vi "Add Port RTM.vi"(8 "error in":errorcluster, 11 "Node Ptr":T1 format="%.0x") -> (0 "error out":errorcluster)   [LabVIEW 2020, in "Ballard ARINC 429 System Explorer.lvlib" / "Implementation.lvlib"]
doc: "This VI runs when the Add Port run-time menu is chosen. It allows the user to create a port with an associated database."
uses:
  Implementation.lvlib
  <vilib>/NI VeriStand/Custom Device Tools/Custom Device Utility Library/Custom Device Utility Library.lvlib
  <vilib>/NI VeriStand/Custom Device API/Custom Device Item Ref.ctl
  <vilib>/NI VeriStand/Custom Device API/Custom Device API.lvlib
  Scripting/Ballard ARINC 429 Scripting.lvlib
  Scripting/Constants.vi
panel:
  in  "Baud Rate":u32
  in  "Database":string(combo)
  in  "Port Name":string
  in  "Help":bool
  in  "Cancel":bool
  in  "OK":bool
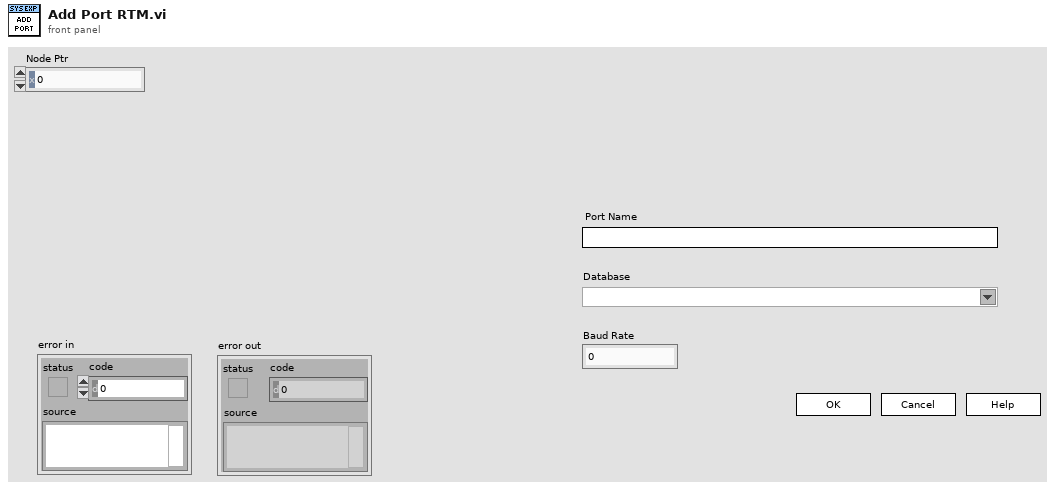
[diagram p1: front panel]
types:
  T1 = typedef "Custom Device API.lvlib/Custom Device Item Ref.ctl" = u64
  T2 = cluster{"Baud Rate":u32, "Port Name":string, "Database Name":string, "Database Path":path, "Databases ref":T1, "Node Ptr":T1}
  T3 = typedef "Ballard ARINC 429 System Explorer.lvlib/Implementation.lvlib/Database.ctl" = cluster{"Baud Rate":u64, "Frames":cluster{"Name":string, "ID":i32}[]}
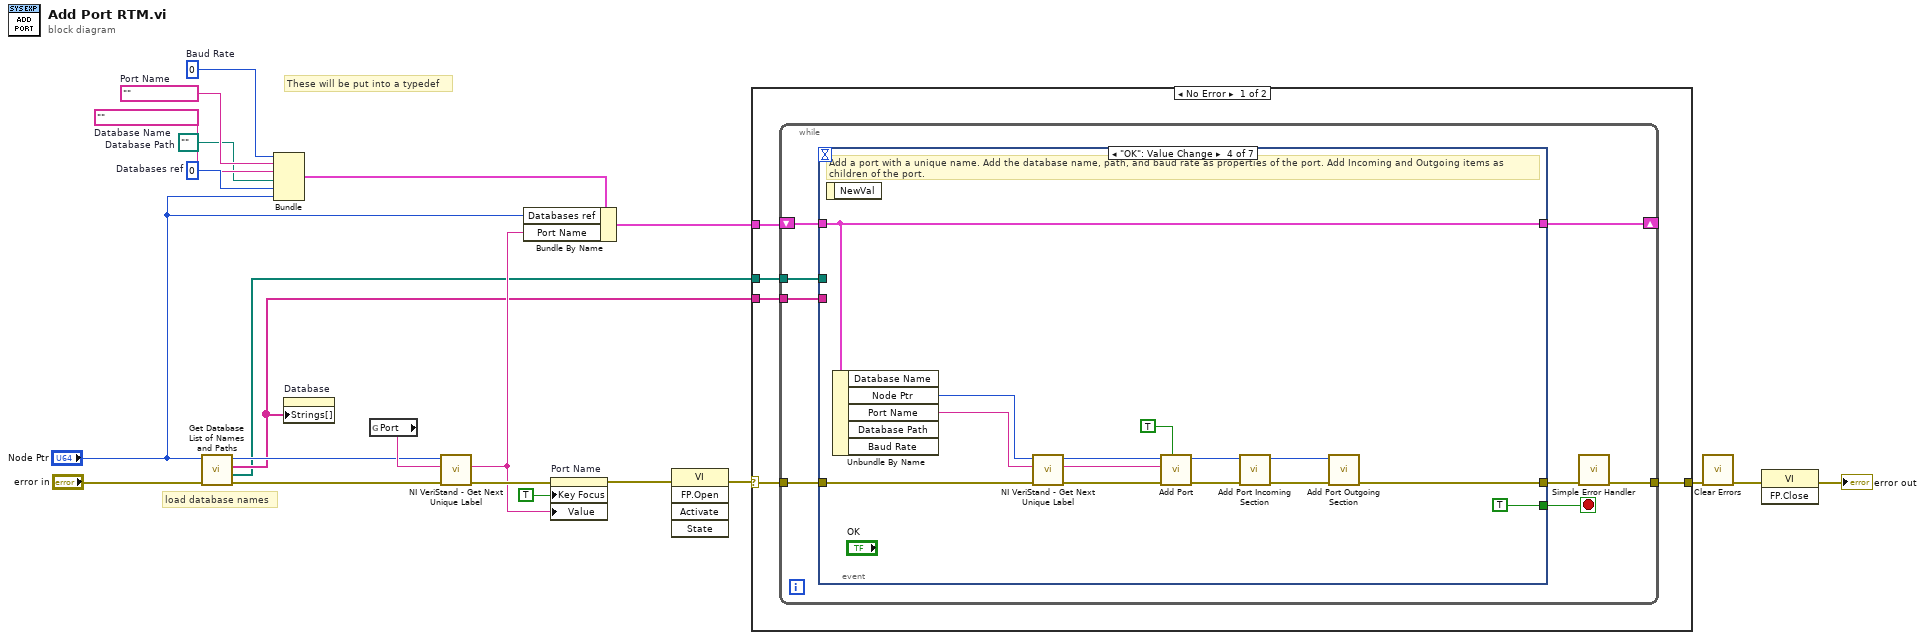
[diagram p0: block diagram]
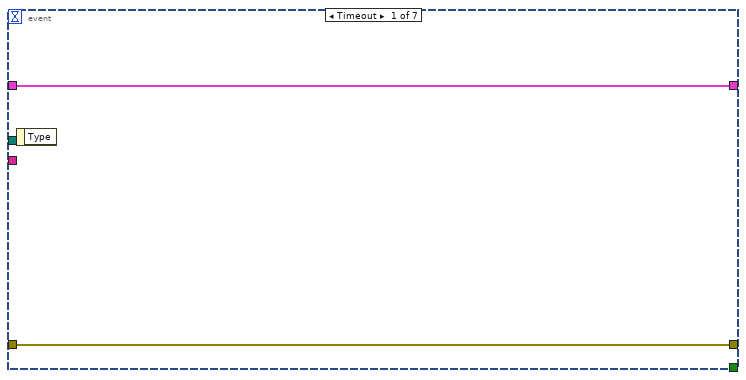
[diagram p2: hidden frame]
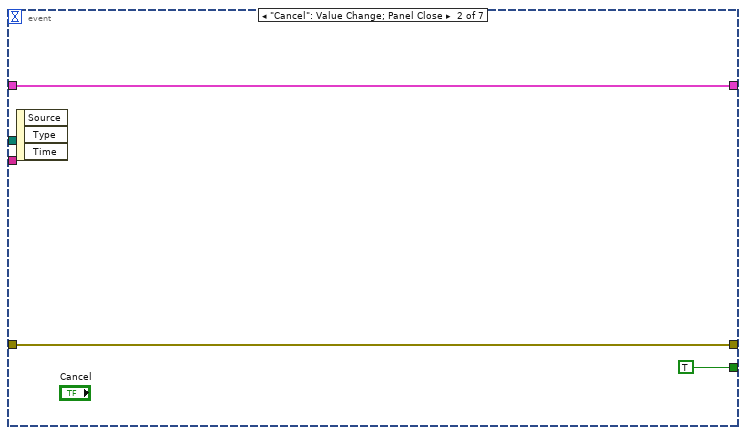
[diagram p3: hidden frame]
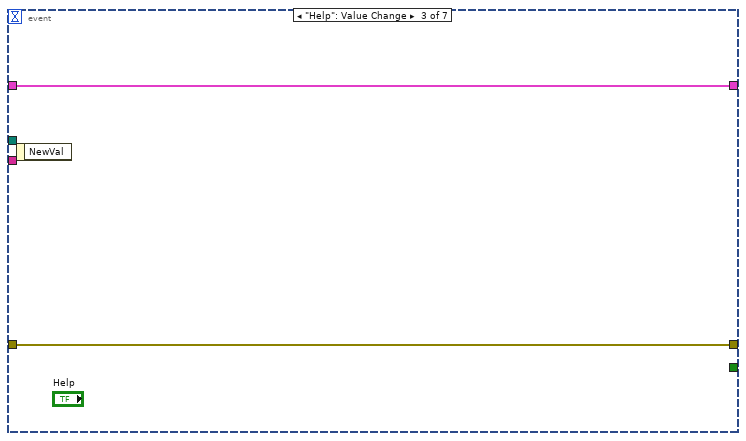
[diagram p4: hidden frame]
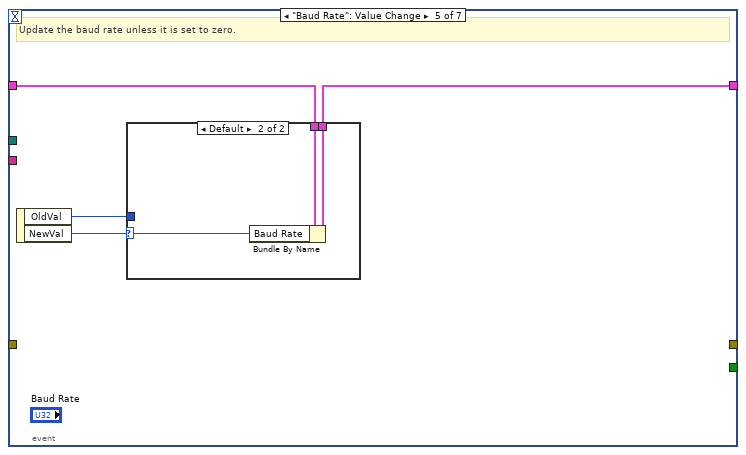
[diagram p5: hidden frame]
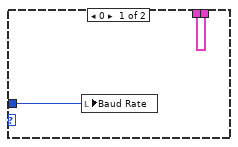
[diagram p6: hidden frame]
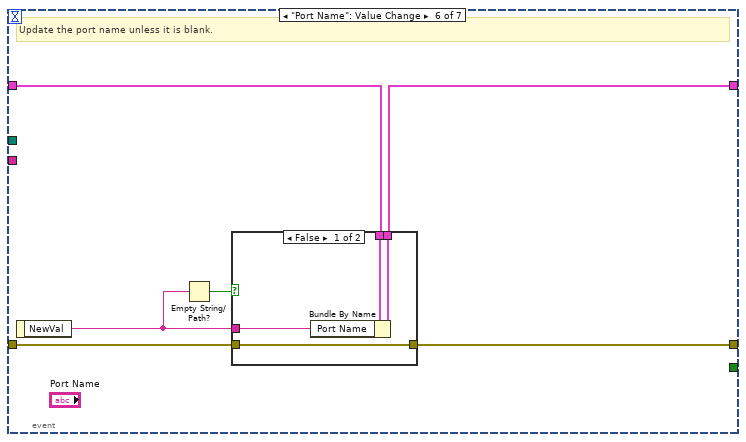
[diagram p7: hidden frame]
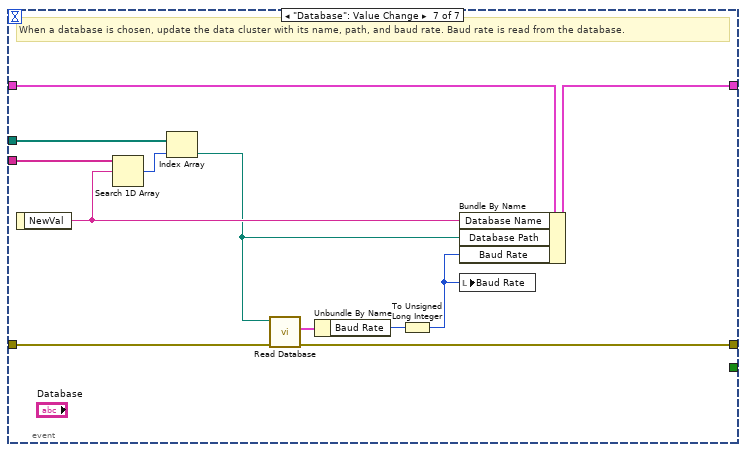
[diagram p9: hidden frame]
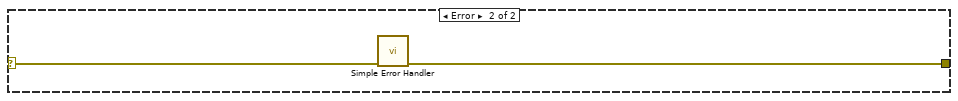
[diagram p10: hidden frame]
diagram:
  w6 = u32 0  # Baud Rate
  w7 = path ""  # Database Path
  w9 = ""  # Database Name
  w12 = T1 0  # Databases ref
  w8 = ""  # Port Name
  # "These will be put into a typedef"
  # "load database names"
  n1 = call "Get Database List of Names and Paths.vi"("error in"="error in", "Databases section Ref"="Node Ptr") -> ("error out"=w4:errorcluster, "Paths"=w1:path[], "Names"=w2:string[], "Databases section Ref out"=w3:T1)  [unwired: 6 in]
  n2 = Bundle("Baud Rate"=w6, "Port Name"=w8, "Database Name"=w9, "Database Path"=w7, "Databases ref"=w12, "Node Ptr"="Node Ptr") -> (w13:T2)  [unwired: 1 in]
  n3 = property on="Database" class="CmbBox"("Strings[]"=w2) -> ()  [unwired: 2 in, 2 out]
  n4 = global read "Constants.vi" "Port"() -> (w14:string)
  n5 = call <vilib>:"NI VeriStand - Get Next Unique Label.vi"("error in (no error)"=w4, "Label"=w14, "Parent Ref in"=w3) -> ("error out"=w15:errorcluster, "Label out"=w11:string)  [unwired: 5 in, 2 out]
  n6 = Bundle By Name(cluster=w13, "Databases ref"="Node Ptr", "Port Name"=w11) -> (w20:T2)
  n7 = property on="Port Name" class="Str"(error in=w15, "Key Focus"=TRUE, "Value"=w11) -> (error out=w19:errorcluster)  [unwired: 1 in, 1 out]
  n8 = invoke class="VI" method="FP.Open"(error in=w19) -> (error out=w18:errorcluster)  [unwired: 4 in, 4 out]
  n9 = case shown="No Error" w18 {
    selector: w18 -> [w27 w91]
    tunnel: [w26 w90] -> w21
    tunnel: w20 -> [w25 _]
    tunnel: w2 -> [w24 _]
    tunnel: w1 -> [w23 _]
    frame No Error {
      n10 = while {
        tunnel: w27 -> [w35]
        tunnel: [w33] -> w26
        shift-right: [w30] -> _
        shift-left: w25 -> [w31]
        tunnel: w24 -> [w29]
        tunnel: w23 -> [w28]
        stop <- w32 stop-if-true
        n11 = event shown="[3] \"OK\": Value Change" {
          selector: _ -> [_ _ _ _ _ _ _]
          dyn-events: _ -> [_ _ _ _ _ _ _]
          timeout: _ -> [_ _ _ _ _ _ _]
          tunnel: [w37 w39 w42 w44 _ w70 w86] -> w34
          tunnel: w35 -> [w37 w39 w42 w55 _ w71 w88]
          tunnel: [_ TRUE ("Discard?") _ TRUE ("Discard?") _ _ _] -> w32
          tunnel: w31 -> [w36 w38 w41 w54 w58 w67 w87]
          tunnel: [w36 w38 w41 w54 w59 w66 w89] -> w30
          tunnel: w29 -> [_ _ _ _ _ _ w81]
          tunnel: w28 -> [_ _ _ _ _ _ w82]
          event Timeout {
            n12 = event-data() -> ()  [unwired: 1 in, 1 out]
          }
          event "Cancel": Value Change; Panel Close {
            n13 = event-data() -> ()  [unwired: 1 in, 3 out]
          }
          event "Help": Value Change {
            n14 = event-data() -> ()  [unwired: 1 in, 1 out]
          }
          event "OK": Value Change {
            # "Add a port with a unique name. Add the database name, path, and baud rate as properties of the port. Add Incoming and Outgoing items as children of the port."
            n15 = event-data() -> ()  [unwired: 1 in, 1 out]
            n16 = Unbundle By Name(w54) -> ("Node Ptr"=w53:T1, "Port Name"=w52:string)  [unwired: 3 out]
            n17 = call <vilib>:"NI VeriStand - Get Next Unique Label.vi"("error in (no error)"=w55, "Label"=w52, "Parent Ref in"=w53) -> ("error out"=w51:errorcluster, "Label out"=w49:string, "Parent Ref dup"=w50:T1)  [unwired: 5 in, 1 out]
            n18 = call "Add Port.vi"("Highlight? (F)"=TRUE, "error in"=w51, "Port Name"=w49, "Incoming Ref"=w50) -> ("error out"=w47:errorcluster, "Port Ref out"=w46:T1)  [unwired: 6 in]
            n19 = call "Add Port Incoming Section.vi"("error in"=w47, "Port Ref"=w46) -> ("error out"=w45:errorcluster, "Port Ref out"=w43:T1)  [unwired: 8 in]
            n20 = call "Add Port Outgoing Section.vi"("error in"=w45, "Port Ref"=w43) -> ("error out"=w44:errorcluster)  [unwired: 8 in, 1 out]
          }
          event "Baud Rate": Value Change {
            # "Update the baud rate unless it is set to zero."
            n21 = event-data() -> ("OldVal"=w57:u32, "NewVal"=w60:u32)  [unwired: 1 in]
            n22 = case shown="Default" w60 {
              selector: w60 -> [_ w63]
              tunnel: w58 -> [w62 w65]
              tunnel: [w62 w64] -> w59
              tunnel: w57 -> [w61 _]
              frame 0 {
                n23 = local write "Baud Rate"(w61) -> ()
              }
              frame Default {
                n24 = Bundle By Name(cluster=w65, "Baud Rate"=w63) -> (w64:T2)
              }
            }
          }
          event "Port Name": Value Change {
            # "Update the port name unless it is blank."
            n25 = event-data() -> ("NewVal"=w68:string)  [unwired: 1 in]
            n26 = Empty String/Path?(string/path=w68) -> (empty?=w69:bool)
            n27 = case shown="False" w69 {
              tunnel: w71 -> [w75 w77]
              tunnel: w68 -> [w73 _]
              tunnel: [w75 w77] -> w70
              tunnel: w67 -> [w74 w76]
              tunnel: [w72 w76] -> w66
              frame False {
                n28 = Bundle By Name(cluster=w74, "Port Name"=w73) -> (w72:T2)
              }
              frame True {
              }
            }
          }
          event "Database": Value Change {
            # "When a database is chosen, update the data cluster with its name, path, and baud rate. Baud rate is read from the database."
            n29 = event-data() -> ("NewVal"=w80:string)  [unwired: 1 in]
            n30 = Search 1D Array(1D array=w81, element=w80) -> (index of element=w83:i32)  [unwired: 1 in]
            n31 = Index Array(array=w82, index=w83) -> (element=w79:path)
            n32 = call "Read Database.vi"("error in"=w88, "Path"=w79) -> ("error out"=w86:errorcluster, "Database"=w85:T3)  [unwired: 8 in]
            n33 = Unbundle By Name(w85) -> ("Baud Rate"=w84:u64)
            n34 = To Unsigned Long Integer(number=w84) -> (unsigned 32bit integer=w78:u32)
            n35 = Bundle By Name(cluster=w87, "Database Name"=w80, "Database Path"=w79, "Baud Rate"=w78) -> (w89:T2)
            n36 = local write "Baud Rate"(w78) -> ()
          }
        }
        n37 = call <vilib>:"Simple Error Handler.vi"("error in (no error)"=w34) -> ("error out"=w33:errorcluster)  [unwired: 4 in, 4 out]
      }
    }
    frame Error {
      n38 = call <vilib>:"Simple Error Handler.vi"("error in (no error)"=w91) -> ("error out"=w90:errorcluster)  [unwired: 4 in, 4 out]
    }
  }
  n39 = call <vilib>:"Clear Errors.vi"("error in (no error)"=w21) -> ("error out"=w17:errorcluster)  [unwired: 5 in, 1 out]
  n40 = invoke class="VI" method="FP.Close"(error in=w17) -> (error out=→"error out":errorcluster)  [unwired: 2 in, 2 out]
